vi "Measure.vi"(6 "error in (no error)":errorcluster, 9 "Tektronix DMM4020 in":refnum<class "Tektronix DMM4020.lvclass">) -> (0 "error out":errorcluster, 2 "Array of Measurement":dbl[](array[numeric]), 3 "Tektronix DMM4020 out":refnum<class "Tektronix DMM4020.lvclass">)   [LabVIEW 2014, in "Generic Digital Multi Meter.lvlib" / "Tektronix DMM4020.lvlib" / "Tektronix DMM4020.lvclass"]
uses:
  Tektronix DMM4020.lvclass
  <instrlib>/Tektronix DMM4020/Tektronix DMM4020.lvlib
  Data Logger/Data Logger.lvclass
panel:
  out "Secondary Display Units":string
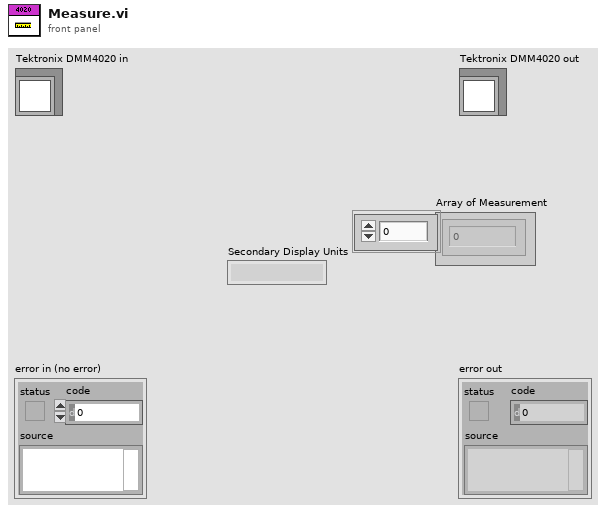
[diagram p1: front panel]
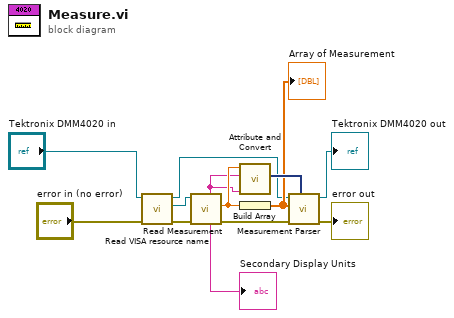
[diagram p0: block diagram]
diagram:
  n1 = call-dynamic "Read VISA resource name.vi"("error in (no error)"="error in (no error)", "Generic Instrument in"="Tektronix DMM4020 in") -> ("error out"=w11:errorcluster, "VISA resource name"=w12:refnum<visa-resource-name>, "Generic Instrument out"=w4:refnum<class "Tektronix DMM4020.lvclass">)  [unwired: 7 in]
  n2 = call <instrlib>:"Read Measurement.vi"("error in (no error)"=w11, "VISA resource name"=w12) -> ("error out"=w2:errorcluster, "Primary Display Measurement"=w8:dbl, "Secondary Display Units"=→"Secondary Display Units":string, "Primary Display Units"=w7:string)  [unwired: 4 in, 2 out]
  n3 = call "Attribute and Convert.vi"("Unit"=w7, "Signal Name"=w7, "Number in"=w8) -> ("Dynamic Signal Out"=w6:dynamicdata)  [unwired: 8 in]
  n4 = Build Array(w8) -> (w5:dbl[])
  "Array of Measurement" <- w5
  n5 = call-dynamic "Measurement Parser.vi"("Waveform Graph"=w6, "error in (no error)"=w2, "Data Array"=w5, "Tektronix DMM4020 in"=w4) -> ("error out"=→"error out":errorcluster, "Tektronix DMM4020 out"=→"Tektronix DMM4020 out":refnum<class "Tektronix DMM4020.lvclass">)  [unwired: 6 in]
